vi "Trigger Files.vi"(11 "2D data":dbl[][](array[numeric]) format="%0.2f") -> ()   [LabVIEW 2011]
uses:
  <vilib>/Utility/file.llb/Write To Spreadsheet File (DBL).vi
panel:
  in  "file path (use dialog)":path
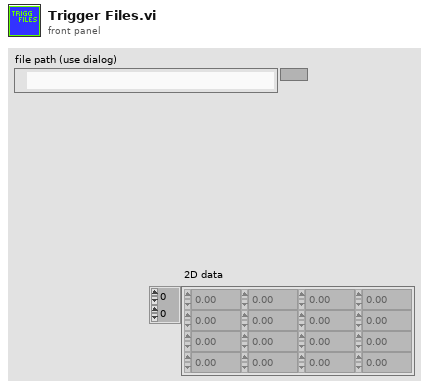
[diagram p1: front panel]
types:
  T1 = enum16{"open", "replace", "create", "open or create", "replace or create", "replace or create with confirmation"}
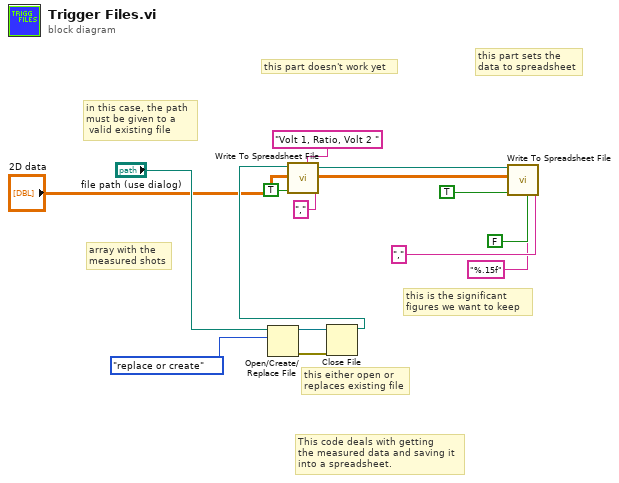
[diagram p0: block diagram]
diagram:
  # "This code deals with getting\nthe measured data and saving it\ninto a spreadsheet."
  # "this is the significant \nfigures we want to keep"
  # "this either open or \nreplaces existing file"
  # "array with the\nmeasured shots"
  # "in this case, the path \nmust be given to a\n valid existing file"
  # "this part sets the \ndata to spreadsheet"
  # "this part doesn't work yet"
  n1 = Open/Create/Replace File(file path (use dialog)="file path (use dialog)", operation (0:open)=T1."replace or create") -> (refnum out=w4:refnum<file>, error out=w3:errorcluster)  [unwired: 4 in, 1 out]
  n2 = Close File(refnum=w4, error in=w3) -> (path=w2:path)  [unwired: 1 out]
  n3 = call-poly <vilib>:"Write To Spreadsheet File.vi"("delimiter (\\t)"="," ("delimiter (\\t)"), "format (%.3f)"="Volt 1, Ratio, Volt 2 ", "append to file? (new file:F)"=TRUE, "file path (dialog if empty)"=w2) -> ("new file path (Not A Path if cancelled)"=w7:path)  [unwired: 4 in]
  n4 = call-poly <vilib>:"Write To Spreadsheet File.vi"("delimiter (\\t)"="," ("delimiter (\\t)"), "transpose? (no:F)"=FALSE, "format (%.3f)"="%.15f", "append to file? (new file:F)"=TRUE, "2D data"="2D data", "file path (dialog if empty)"=w7) -> ()  [unwired: 2 in, 1 out]
